vi "set values for a control in a cluster using reference.vi"(8 "value":variant, 10 "name":string, 11 "Clust Refnum":refnum<vi>) -> ()   [LabVIEW 2015]
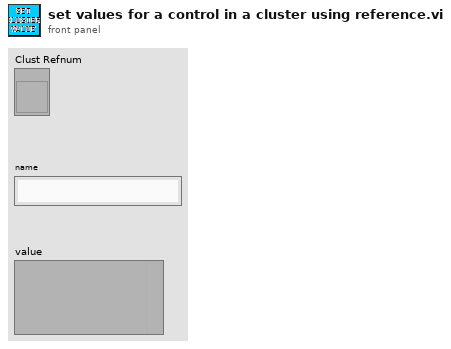
[diagram p1: front panel]
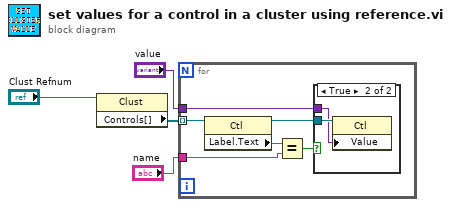
[diagram p0: block diagram]
diagram:
  n1 = property class="Clust"(reference="Clust Refnum") -> ("Controls[]"=w3:refnum<vi>[])  [unwired: 1 in, 2 out]
  n2 = for {
    tunnel: w3 -> [w10] mode=indexing
    tunnel: "name" -> [w8]
    tunnel: "value" -> [w5]
    n3 = property class="Ctl"(reference=w10) -> (reference out=w6:refnum<vi>, "Label.Text"=w9:string)  [unwired: 1 in, 1 out]
    n4 = Equal?(x=w9, y=w8) -> (x = y?=w7:bool)
    n5 = case shown="True" w7 {
      tunnel: w6 -> [_ w12]
      tunnel: w5 -> [_ w11]
      frame False {
      }
      frame True {
        n6 = property class="Ctl"(reference=w12, "Value"=w11) -> ()  [unwired: 1 in, 2 out]
      }
    }
  }
